vi "get_context.vi"(8 "error in (no error)":errorcluster, 11 "WebSocket Queue Logger in":refnum<class "WebSocket Queue Logger.lvclass">) -> (0 "error out":errorcluster, 1 "remote address":string, 2 "remote port":u16, 3 "WebSocket Queue Logger out":refnum<class "WebSocket Queue Logger.lvclass">)   [LabVIEW 2019, in "WebSocket Server Toolkit.lvlib" / "WebSocket Queue Logger.lvclass"]
uses:
  WebSocket Queue Logger.lvclass
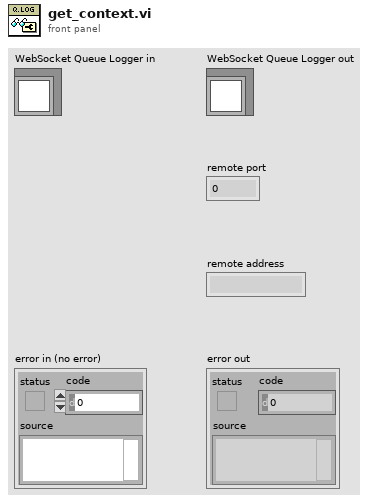
[diagram p1: front panel]
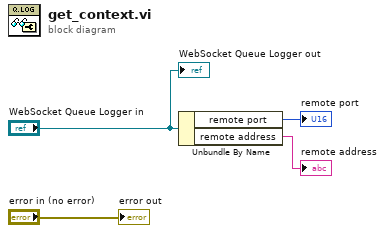
[diagram p0: block diagram]
diagram:
  n1 = Unbundle By Name("WebSocket Queue Logger in") -> ("remote port"=→"remote port":u16, "remote address"=→"remote address":string)
  "error out" <- "error in (no error)"
  "WebSocket Queue Logger out" <- "WebSocket Queue Logger in"
